vi "ReversedEngineering UpdateAttributes.vi"(1 "ClassPath/LvClassRef":variant, 2 "NewAttributes":string="Sträng:STRING\nMittCluster:CLUSTER", 3 "ClassInfo":cluster{"ClassNamn":string, "ClassPath":path}[](array[cluster]), 5 "error in (no error)":errorcluster, 6 "Don't Prompt (False)":bool, 7 "Attributes":T1[](array[typedef]), 8 "Stereotype":string) -> (18 "Cancel":bool=TRUE, 19 "error out":errorcluster)   [LabVIEW 2012] (continued)
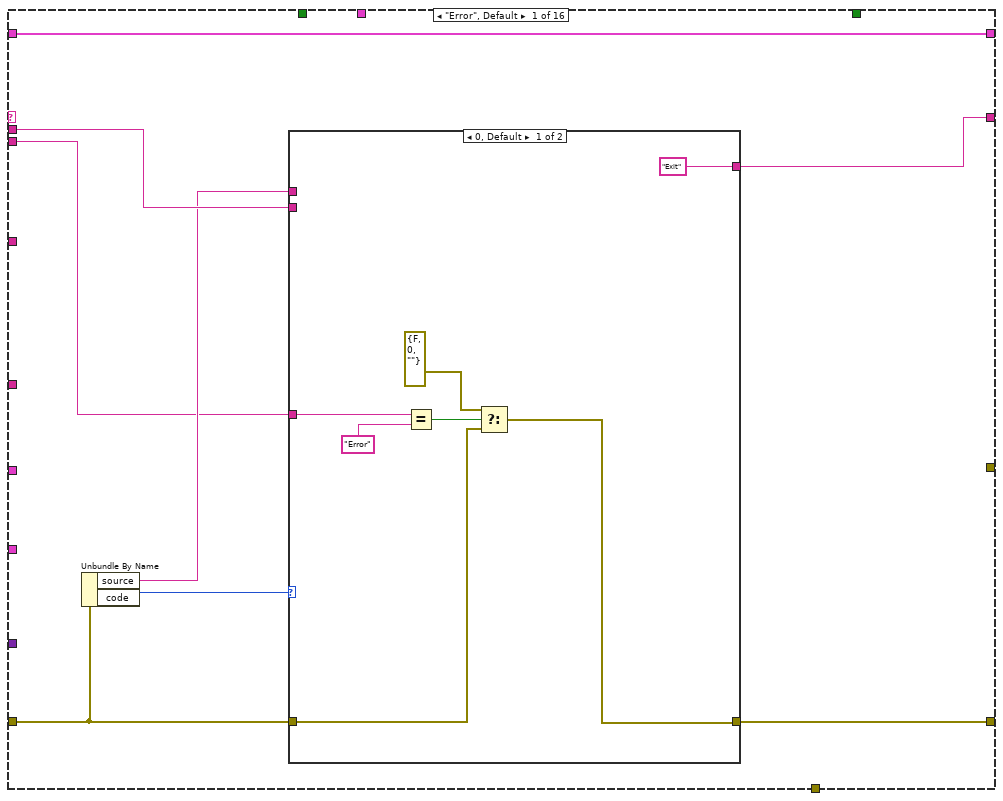
[diagram p3: hidden frame]
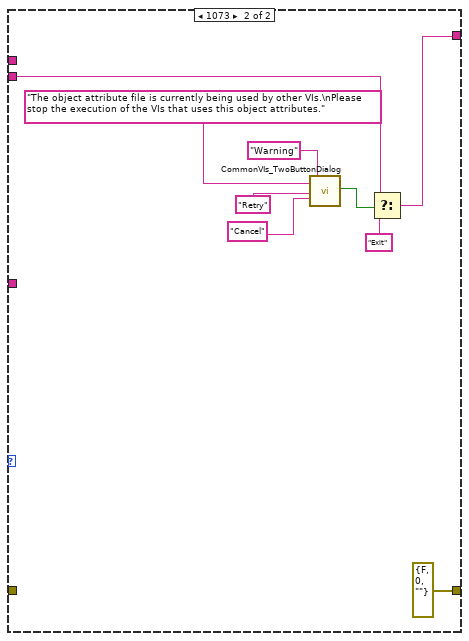
[diagram p4: hidden frame]
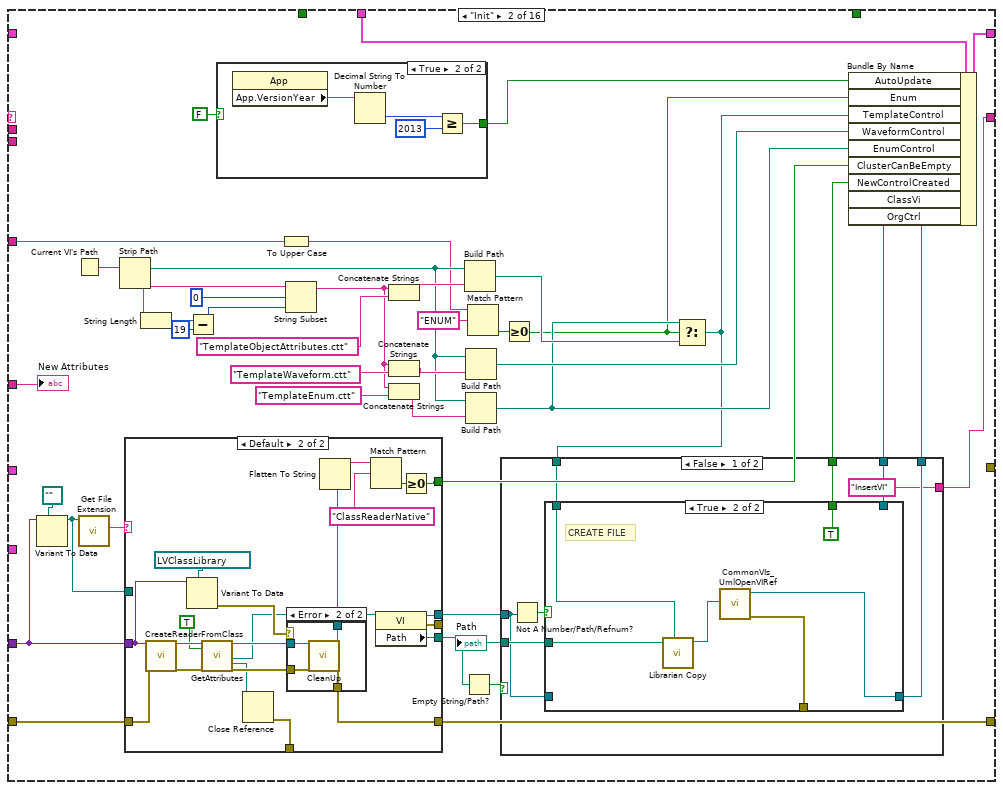
[diagram p5: hidden frame]
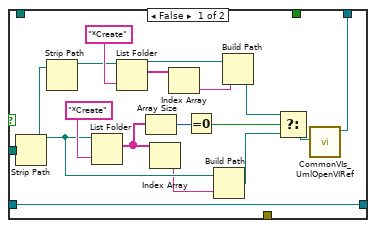
[diagram p7: hidden frame]
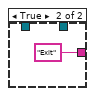
[diagram p8: hidden frame]
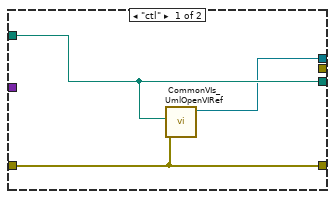
[diagram p9: hidden frame]
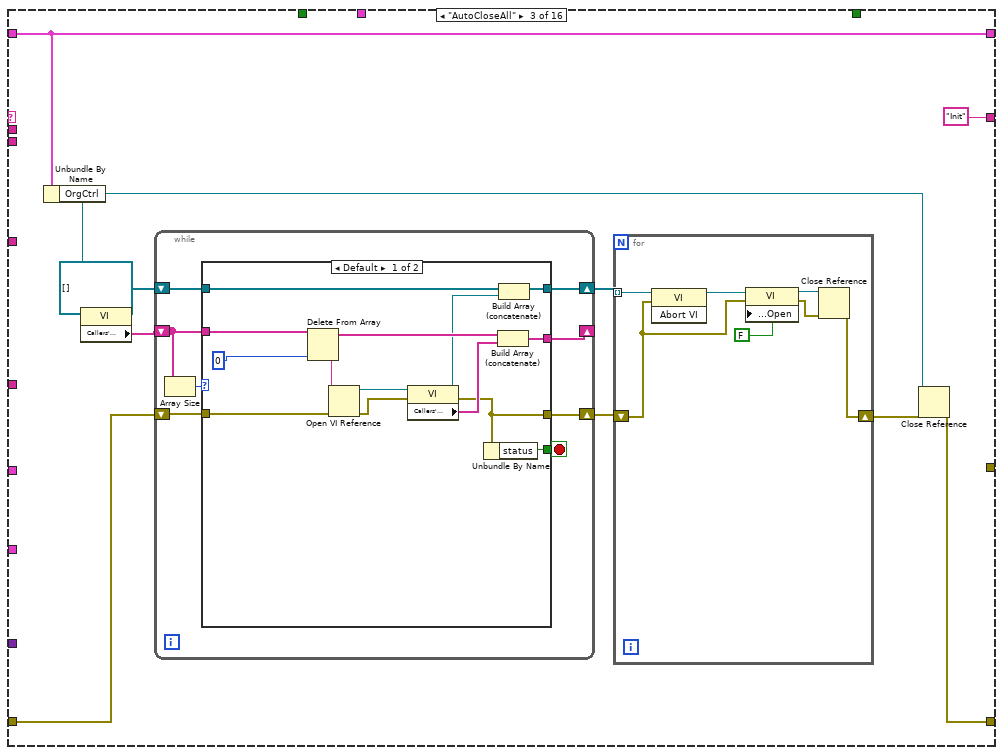
[diagram p11: hidden frame]
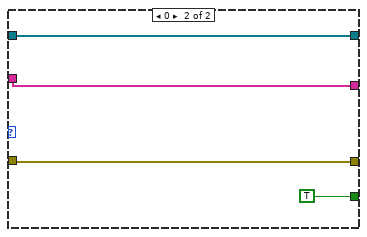
[diagram p12: hidden frame]
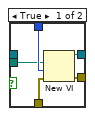
[diagram p13: hidden frame]
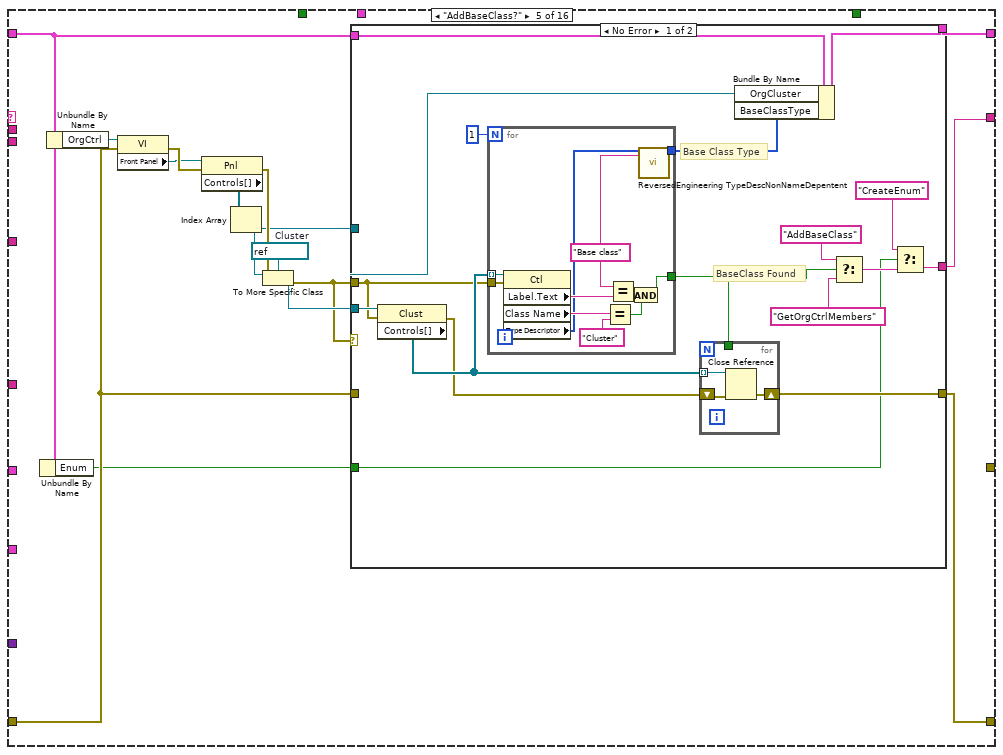
[diagram p15: hidden frame]
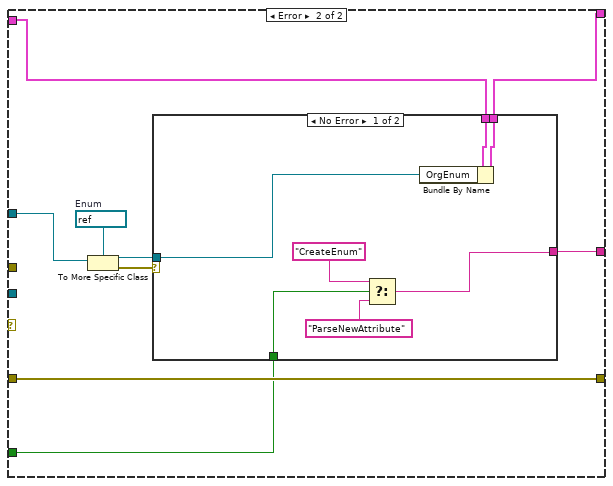
[diagram p16: hidden frame]
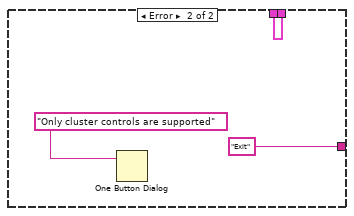
[diagram p17: hidden frame]
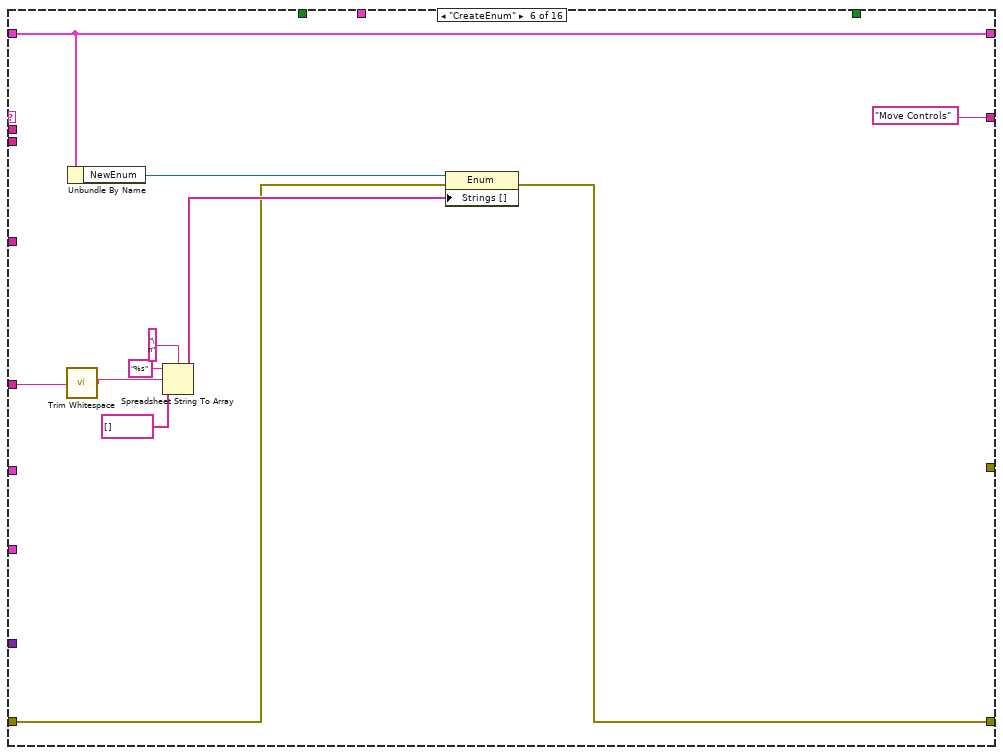
[diagram p18: hidden frame]
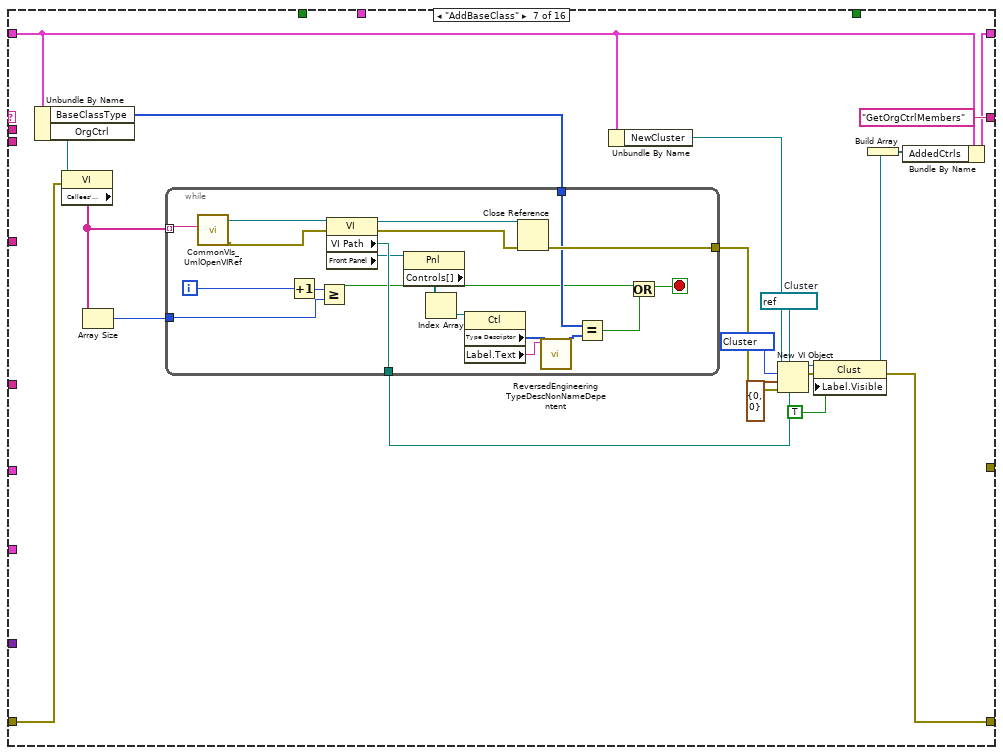
[diagram p19: hidden frame]
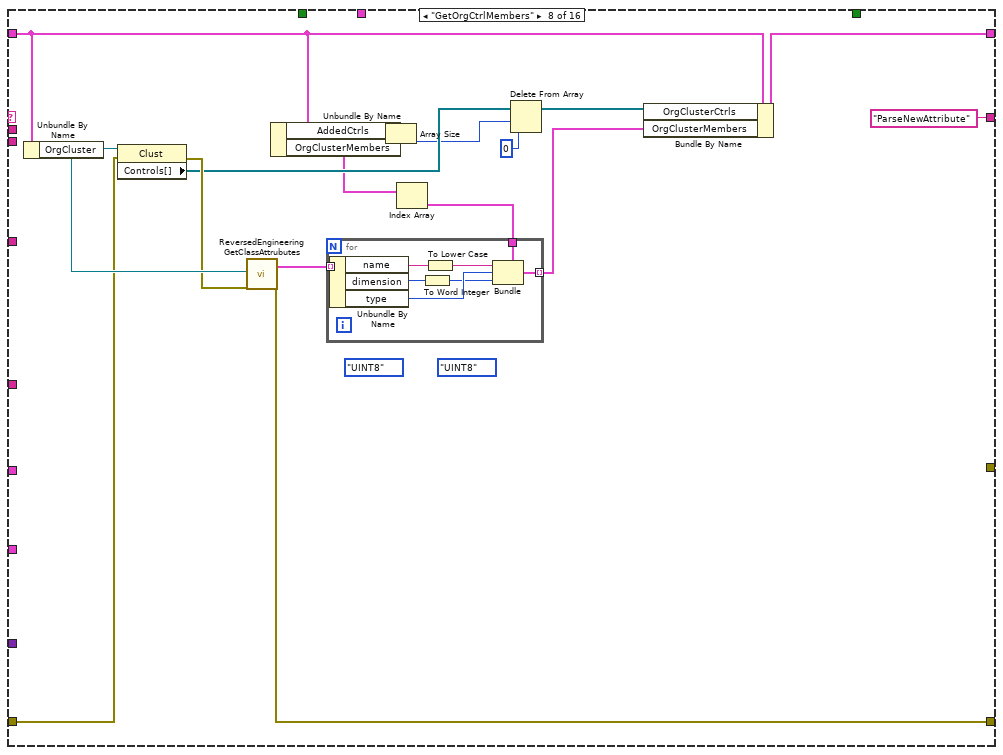
[diagram p20: hidden frame]
"Pressure Tank"=21753, "Pressure Tank 1"=3075, "Preview Queue Element"=9112, "Printable?"=1124, "Priority Queue Refnum"=3425, "Property Node"=1920, "Pulldown Menu Ring"=3061, "Push Button"=21001, "Queue Refnum"=3474, "Queue Refnum 1"=3424, "Quit LabVIEW"=1352, "Quotient & Remainder"=1056, "RT FIFO Create"=24000, "RT FIFO Delete"=24003, "RT FIFO Read"=24001, "RT FIFO Write"=24002, "Radio Buttons"=22001, "Raised Box"=3637, "Raised Box 1"=3600, "Raised Circle"=3603, "Raised Down Triangle"=3615, "Raised Frame"=3606, "Raised Left Triangle"=3612, "Raised Right Triangle"=3613, "Raised Rounded Box"=3609, "Raised Up Triangle"=3614, "Random Number (0-1)"=1070, "RcvRespMsg"=1972, "Re/Im To Complex"=1046, "Re/Im To Polar"=23060, "Read Datalog"=8069, "Read Device"=1432, "Read File"=1407, "Read from Binary File"=8051, "Read from Text File"=8070, "ReadStatus"=1973, "Receive"=1974, "ReceiveSetup"=1975, "Recessed Box"=3601, "Recessed Circle"=3604, "Recessed Down Triangle"=3619, "Recessed Frame"=3607, "Recessed Left Triangle"=3616, "Recessed Menu Ring"=3019, "Recessed Right Triangle"=3617, "Recessed Rounded Box"=3610, "Recessed Up Triangle"=3618, "Reciprocal"=1059, "Reciprocal Of Pi"=23507, "Reciprocal Of e"=23511, "Rectangular Stop Button"=3128, "Refnum to Path"=1424, "Refnum to Session"=2306, "Register Event Callback"=2078, "Register For Events"=2065, "Register Session"=2319, "Release Notifier"=9102, "Release Queue"=9109, "Replace Array Subset"=3910, "Replace Substring"=3913, "Request Deallocation"=1610, "ResetSys"=1976, "Reshape Array"=2055, "Reverse 1D Array"=1900, "Reverse String"=1537, "Right Arrow"=3825, "Right Bow Valve"=21765, "Right Bow Valve 1"=3805, "Right Bow Valve 2"=3705, "Right Down Elbow"=3717, "Right Down Elbow 1"=3817, "Right Pump"=3819, "Right Pump 1"=3719, "Right Rect Valve"=3704, "Right Rect Valve 1"=3804, "Right Rect Valve 2"=21764, "Right Tee"=3815, "Right Tee 1"=3715, "Right Up Elbow"=3714, "Right Up Elbow 1"=3814, "Ring Constant"=2008, "Rocker"=21002, "Rotary Feeder"=3830, "Rotate"=1082, "Rotate 1D Array"=1906, "Rotate Left With Carry"=1606, "Rotate Right With Carry"=1607, "Rotate String"=1536, "Round Button"=3100, "Round LED"=3120, "Round LED 1"=21012, "Round Light"=3104, "Round Push Button"=3112, "Round Push Button 2"=3118, "Round Radio Button"=3106, "Round Stop Button"=3127, "Round To +Infinity"=1076, "Round To -Infinity"=1075, "Round To Nearest"=1055, "Rydberg Constant (1/m)"=23521, "Scale By Power Of 2"=1074, "Scan From File"=2082, "Scan From String"=2080, "Scan String For Tokens"=8101, "Scan Value"=1534, "Search 1D Array"=1901, "Search and Replace String"=3914, "Search/Split String"=1538, "Secant"=1203, "Seconds To Date/Time"=1309, "Seek"=1409, "Select"=1516, "Send"=1977, "Send Notification"=9104, "SendCmds"=1978, "SendDataBytes"=1979, "SendIFC"=1980, "SendLLO"=1982, "SendList"=1981, "SendSetup"=1983, "Session to Refnum"=2307, "Set Datalog Position"=8072, "Set File Position"=8073, "Set File Size"=8074, "Set Menu Item Info"=9006, "Set Number of Records"=8075, "Set Occurrence"=1702, "Set Permissions"=8076, "Set Type and Creator"=8077, "Set Variant Attribute"=8204, "Set Waveform Attribute"=8207, "SetRWLS"=1984, "SetTimeOut"=1985, "Shared Variable Constant"=3473, "Shared Variable Control"=21814, "Shared Variable Control 1"=3472, "Shared Variable to String"=1831, "Sign"=1049, "Simple Horizontal Slide"=3003, "Simple Numeric"=3029, "Simple Numeric 1"=2900, "Simple String"=2115, "Simple Vertical Slide"=3002, "Simulation Loop"=2099, "Sinc"=1227, "Sine"=1200, "Sine & Cosine"=1220, "Size Handle"=1603, "Slide Switch"=21011, "Sort 1D Array"=1120, "Sort Array of String, Sort Array of String 1"=23065, "Speed Of Light In Vacuum (m/sec)"=23518, "Split 1D Array"=1908, "Split Button"=21020, "Split Number"=1170, "Split Signals"=2351, "Spreadsheet String To Array"=1539, "Square"=23059, "Square Button"=3101, "Square LED"=3121, "Square LED 1"=21013, "Square Light"=3105, "Square Push Button"=3113, "Square Push Button 2"=3119, "Square Radio Button"=3107, "Square Root"=1060, "Stacked Sequence Structure"=2000, "State Diagram"=2051, "Static VI Reference"=2084, "Stop"=1350, "Stop Button"=21230, "String Constant"=2007, "String Control"=21701, "String Control 1"=3200, "String Indicator"=21702, "String Indicator 1"=3201, "String Length"=1502, "String Subset"=1503, "String To Byte Array"=1608, "String To IP"=1711, "String To Path"=1078, "String to Shared Variable"=1830, "Strip Path"=1420, "SubPanel"=21810, "SubPanel (Classic)"=21811, "Subtract"=3916, "Subtract 1"=1051, "Swap Bytes"=1162, "Swap Values"=2401, "Swap Vector Element"=1912, "Swap Words"=1163, "System Button"=3130, "System Cancel Button"=3131, "System Checkbox"=3132, "System Chiseled Line"=3632, "System Colored Rectangle"=3625, "System Combo Box"=21917, "System Enum"=3062, "System Horizontal Pointer Slide"=21902, "System Horizontal Progress Bar"=21910, "System Horizontal Slide"=21904, "System Label"=21961, "System Listbox"=21805, "System Multicolumn Listbox"=21798, "System Numeric"=21919, "System Path Control"=21922, "System Pict Ring"=21925, "System Radio Button"=3133, "System Radio Buttons"=22002, "System Recessed Frame"=3624, "System Ring"=3060, "System Spin Control"=21900, "System String"=21920, "System Tab Control"=3331, "System Table"=21797, "System Time Stamp"=21967, "System Tree"=21794, "System Vertical Pointer Slide"=21901, "System Vertical Progress Bar"=21909, "System Vertical Slide"=21903, "TCP Close Connection"=1713, "TCP Create Listener"=1717, "TCP Flattened Read"=1718, "TCP Flattened Write"=1719, "TCP Flex Read"=1720, "TCP Flex Write"=1721, "TCP Network Connection Refnum"=3407, "TCP Open Connection"=1715, "TCP Read"=1716, "TCP Wait On Listener"=1712, "TCP Write"=1714, "TDMS Close"=2013, "TDMS Defragment"=2019, "TDMS File"=3477, "TDMS Flush"=2017, "TDMS Get Properties"=2015, "TDMS List Contents"=2016, "TDMS Open"=2012, "TDMS Read"=2011, "TDMS Set Properties"=2014, "TDMS Write"=2010, "TDMS Write IP"=2018, "Tab Constant"=23502, "Tab Control"=3332, "Tab Control 1"=3330, "Table"=21796, "Table 1"=21790, "Tag Attribute Ring"=2063, "Tag Constant"=2089, "Tag Control"=3302, "Tag Control 1"=21742, "Tag Indicator"=3303, "Tag Indicator 1"=21743, "Tangent"=1202, "Tank"=21006, "Tank 1"=3020, "Temporary Directory"=1435, "TestSRQ"=1986, "TestSys"=1987, "Text & Pict Ring"=21603, "Text & Pict Ring 1"=3016, "Text Button"=21015, "Text Ring"=21601, "Text Ring 1"=3014, "Text to UTF-8"=23066, "Thermometer"=21007, "Thermometer 1"=3021, "Thick Chiseled Line"=3630, "Thick Line"=3629, "Thick Line with Arrow"=3631, "Thick Lowered Box"=3635, "Thin Chiseled Line"=3627, "Thin Line"=3626, "Thin Line with Arrow"=3628, "Threshold 1D Array"=1909, "Tick Count (ms)"=1300, "Time Stamp Constant"=2068, "Time Stamp Control"=5555, "Time Stamp Control 1"=21913, "Time Stamp Indicator"=5556, "Time Stamp Indicator 1"=21914, "Timed Loop"=5570, "Timed Sequence"=5573, "To Byte Integer"=1140, "To Double Precision Complex"=1152, "To Double Precision Float"=1147, "To Extended Precision Complex"=1154, "To Extended Precision Float"=1149, "To Long Integer"=1142, "To Lower Case"=1189, "To More Generic Class"=8017, "To More Specific Class"=8016, "To OLE Variant"=8002, "To Quad Integer"=1155, "To Single Precision Complex"=1151, "To Single Precision Float"=1146, "To Time Stamp"=5560, "To Unsigned Byte Integer"=1143, "To Unsigned Long Integer"=1145, "To Unsigned Quad Integer"=1156, "To Unsigned Word Integer"=1144, "To Upper Case"=1188, "To Variant"=8201, "To Word Integer"=1141, "Traditional DAQ Channel"=21733, "Traditional DAQ Channel 1"=3320, "Traditional DAQ Channel 2"=2085, "Transpose 2D Array"=1902, "Tree"=21819, "Tree 1"=21793, "Trigger"=1988, "TriggerList"=1989, "Two Button Dialog"=1341, "Type Cast"=1166, "Type and Creator"=1434, "UDP Close"=1726, "UDP Multicast Open"=1727, "UDP Network Connection Refnum"=3418, "UDP Open"=1723, "UDP Read"=1724, "UDP Write"=1725, "UTF-8 to Text"=23067, "Unbundle"=2048, "Unbundle By Name"=2058, "Unflatten From String"=1165, "Unflatten From XML"=8401, "Unpackage Matrix"=23000, "Unregister For Events"=2076, "Unregister Session"=2320, "Up Arrow"=3823, "Up Bow Valve"=21763, "Up Bow Valve 1"=3803, "Up Bow Valve 2"=3703, "Up Rect Valve"=3702, "Up Rect Valve 1"=3802, "Up Rect Valve 2"=21762, "Up Tee"=3712, "Up Tee 1"=3812, "User Defined Refnum"=3428, "User Defined Refnum Tag"=3429, "User Defined Refnum Tag 1"=21745, "User Defined Refnum Tag Flatten"=3454, "User Defined Refnum Tag Flatten 1"=21747, "User Defined Tag"=2114, "User Defined Tag 1"=21749, "User Item"=3506, "VI Library"=1425, "VI Refnum"=3422, "VI Server Reference"=2091, "VISA Assert Interrupt Signal"=2309, "VISA Assert Trigger"=1929, "VISA Assert Utility Signal"=2310, "VISA Clear"=1927, "VISA Close"=1922, "VISA Disable Event"=1940, "VISA Discard Events"=1941, "VISA Enable Event"=1942, "VISA Find Resource"=1923, "VISA Flush I/O Buffer"=2302, "VISA GPIB Command"=2315, "VISA GPIB Control ATN"=2316, "VISA GPIB Control REN"=2304, "VISA GPIB Pass Control"=2317, "VISA GPIB Send IFC"=2318, "VISA In 16"=1930, "VISA In 32"=1944, "VISA In 8"=1936, "VISA Lock"=1993, "VISA Map Address"=1932, "VISA Map Trigger"=2311, "VISA Memory Allocation"=1997, "VISA Memory Free"=1998, "VISA Move"=2303, "VISA Move In 16"=1948, "VISA Move In 32"=1991, "VISA Move In 8"=1946, "VISA Move Out 16"=1949, "VISA Move Out 32"=1992, "VISA Move Out 8"=1947, "VISA Open"=2308, "VISA Out 16"=1931, "VISA Out 32"=1945, "VISA Out 8"=1937, "VISA Peek 16"=1934, "VISA Peek 32"=1995, "VISA Peek 8"=1938, "VISA Poke 16"=1935, "VISA Poke 32"=1996, "VISA Poke 8"=1939, "VISA Read"=1925, "VISA Read STB"=1928, "VISA Read To File"=2313, "VISA Refnum to Session"=2300, "VISA Resource Name"=21737, "VISA Resource Name 1"=3421, "VISA Set I/O Buffer Size"=2301, "VISA Status Description"=1924, "VISA USB Control In"=2086, "VISA USB Control Out"=2087, "VISA Unlock"=1994, "VISA Unmap Address"=1933, "VISA Unmap Trigger"=2312, "VISA VXI Cmd or Query"=2305, "VISA Wait on Event"=1943, "VISA Write"=1926, "VISA Write From File"=2314, "VISA resource name"=3409, "Variant"=3310, "Variant To Data"=8003, "Variant To Flattened String"=8203, "Vert Line"=3822, "Vert Pipe"=3716, "Vert Pipe 1"=3816, "Vert Rocker"=21740, "Vertical Fill Slide"=21014, "Vertical Fill Slide 1"=3009, "Vertical Graduated Bar"=21107, "Vertical Pointer Slide"=21017, "Vertical Pointer Slide 1"=3007, "Vertical Progress Bar"=21104, "Vertical Scrollbar"=21111, "Vertical Slide"=3004, "Vertical Slide Switch"=21741, "Vertical Slide Switch 1"=3115, "Vertical Smooth Box"=3634, "Vertical Splitter Bar"=21860, "Vertical Splitter Bar (Classic)"=21862, "Vertical Splitter Bar (System)"=21864, "Vertical Switch"=3109, "Vertical Toggle Switch"=21005, "Vertical Toggle Switch 1"=3111, "Volume Info"=1414, "Wait (ms)"=1302, "Wait For Activity"=1722, "Wait For Front Panel Activity"=1328, "Wait Until Next ms Multiple"=1327, "Wait for GPIB RQS"=1952, "Wait on Notification"=9105, "Wait on Notification from Multiple"=9106, "Wait on Occurrence"=1701, "WaitSRQ"=1990, "Waveform Chart"=3501, "Waveform Chart 1"=21717, "Waveform Chart 2"=21010, "Waveform Graph"=21703, "Waveform Graph 1"=3504, "While Loop"=2003, "While Loop 1"=2352, "White Space?"=1125, "Write Datalog"=8079, "Write Device"=1431, "Write File"=1408, "Write to Binary File"=8078, "Write to Text File"=8080, "XY Graph"=3500, "XY Graph 1"=21716, "Xmath Script Node"=9022, "Y-th root of X"=23062]
                      (unwired) refnum<vi> refnum  # LVObjectRefNum
                      n229 = New VI Object(vi object class=w701, owner refnum=w707, style=w702, position/next to=w706, 8:w704) -> (object refnum=w703:refnum<vi>, 0:w705:errorcluster)  [unwired: 3 out]
                    }
                  }
                  n230 = case shown="0, Default" w527 {
                    tunnel: w530 -> [w540 w543]
                    tunnel: [w540 w542] -> w528
                    tunnel: w526 -> [_ w542]
                    tunnel: [_ w541] -> _
                    frame 0, Default {
                    }
                    frame 1.. {
                      n231 = Close Reference(reference=w543) -> (error out=w541:errorcluster)  [unwired: 1 in]
                    }
                  }
                }
                frame True {
                  # "Control exists, no change, just copy"
                  n232 = Index Array(array=w746, index=w711) -> (element=w724:refnum<vi>)
                  n233 = property class="Ctl"(reference=w744, error in=w727) -> ("Position:Top"=w743:i32, "Bounds:Height"=w742:u32)  [unwired: 2 out]
                  n234 = property on="Panel" class="VI"(reference=w733, error in=w727) -> (error out=w734:errorcluster, "Front Panel"=w728:refnum<vi>)  [unwired: 1 out]
                  n235 = Build Array (concatenate)(w712, w711) -> (w710:i32[])
                  n236 = Add(x=w743, y=w742) -> (x+y=w741:u32)
                  n237 = property on="Select" class="Ctl"(reference=w724, error in=w734, "Selected"=TRUE) -> (error out=w735:errorcluster)  [unwired: 1 out]
                  n238 = Increment(x=w741) -> (x+1=w740:u32)
                  n239 = Bundle("element"=u32 0, w740) -> (w720:cluster{"element":u32, u32})  [unwired: 1 out]
                  n240 = invoke on="Copy" class="Pnl" method="Copy Selection"(reference=w728, error in=w735) -> (reference out=w737:refnum<vi>, error out=w736:errorcluster)  [unwired: 1 in, 1 out]
                  n241 = Close Reference(reference=w737, error in (no error)=w736) -> (error out=w726:errorcluster)
                  n242 = property on="Select" class="Ctl"(reference=w724, error in=w726, "Selected"=FALSE) -> (error out=w725:errorcluster)  [unwired: 1 out]
                  n243 = property on="Panel" class="VI"(reference=w723, error in=w725) -> (error out=w745:errorcluster, "Front Panel"=w719:refnum<vi>)  [unwired: 1 out]
                  n244 = invoke class="Pnl" method="Paste Selection"(reference=w719, error in=w745, "Pos"=cluster{"Left":i32, "Top":i32} {"Left"=50, "Top"=50}) -> (reference out=w716:refnum<vi>, error out=w715:errorcluster)  [unwired: 2 in, 3 out]
                  n245 = property on="Panel" class="Pnl"(reference=w716, error in=w715) -> (reference out=w730:refnum<vi>, error out=w714:errorcluster, "Controls[]"=w731:refnum<vi>[])
                  n246 = Delete From Array(array=w731) -> (deleted portion=w709:refnum<vi>, array with subset deleted=w718:refnum<vi>[])  [unwired: 2 in]
                  n247 = invoke class="Ctl" method="Move"(reference=w709, error in=w714, "position"=w720, "owner"=w721) -> (reference out=w708:refnum<vi>, error out=w713:errorcluster)  [unwired: 2 in, 4 out]
                  n248 = invoke on="Paste" class="Ctl" method="Update Typedef"(reference=w709) -> ()  [unwired: 2 in, 3 out]
                  n249 = Close Reference(reference=w730, error in (no error)=w713) -> (error out=w729:errorcluster)
                  n250 = for {
                    tunnel: w718 -> [w747] mode=indexing
                    tunnel: w708 -> [_]
                    n251 = Close Reference(reference=w747) -> ()  [unwired: 1 in, 1 out]
                  }
                  n252 = invoke on="EmptyClip" class="App" method="Clipboard.Empty"(error in=w729) -> (error out=w732:errorcluster)  [unwired: 2 in, 2 out]
                }
              }
              n253 = property class="Ctl"(reference=w512, error in=w520, "Label.Text"=w492, "Auto-Update From Typedef"=TRUE ("Label.Visible")) -> (reference out=w522:refnum<vi>, error out=w521:errorcluster)
              n254 = property class="Ctl"(reference=w522, error in=w521, "Label.Text"=w492, "Label.Visible"=TRUE) -> (reference out=w523:refnum<vi>, error out=w519:errorcluster)
            }
            n255 = Array Size(array=w466) -> (size(s)=w465:i32)
            n256 = Array Size(array=w467) -> (size(s)=w464:i32)
            n257 = Equal?(x=w465, y=w464) -> (x = y?=w463:bool)
            n258 = And Array Elements(Boolean array=w467) -> (logical AND=w468:bool)
            n259 = And(x=w463, y=w468) -> (x .and. y?=w462:bool)
            n260 = Build Array (concatenate)(w482, w480) -> (w481:refnum<vi>[])
            n261 = Bundle By Name(cluster=w471, "NoUpdate"=w462, "AddedCtrls"=w481) -> (w483:T4)
          }
          frame "Move Controls" {
            n262 = Unbundle By Name(w753) -> ("NewCtrl"=w764:refnum<vi>, "NewCluster"=w763:refnum<vi>, "OrgCtrl"=w760:refnum<vi>, "OrgCluster"=w761:refnum<vi>, "NewEnum"=w754:refnum<vi>)
            n263 = property class="VI"(reference=w760) -> ("Front Panel Window:Origin"=w762:T12)  [unwired: 1 in, 2 out]
            n264 = property class="VI"(reference=w764) -> ("Front Panel Window:Origin"=w755:T12)  [unwired: 1 in, 2 out]
            n265 = property class="Clust"(reference=w761, "Position"=w762) -> ()  [unwired: 1 in, 2 out]
            n266 = property class="Clust"(reference=w763, "Position"=w755) -> ()  [unwired: 1 in, 2 out]
            n267 = property class="Enum"(reference=w754, "Position"=w755) -> ()  [unwired: 1 in, 2 out]
            n268 = case shown="True" FALSE {
              tunnel: [_ w766] -> w749
              frame False {
              }
              frame True {
                n269 = property class="App"() -> ("App.VersionYear"=w769:string)  [unwired: 2 in, 2 out]
                n270 = Decimal String To Number(string=w769) -> (number=w768:i32)  [unwired: 2 in, 1 out]
                n271 = Greater Or Equal?(x=w768, y=2013) -> (x >= y?=w766:bool)
              }
            }
            n272 = Unbundle By Name(w753) -> ("NoUpdate"=w751:bool, "AutoUpdate"=w750:bool)
            n273 = Compound Arithmetic op=OR(w756, w751, w750, w749) -> (w752:bool)
            n274 = Select(t="SaveCtrl" ("y"), s=w752, f="Idle" ("y")) -> (s? t:f=w757:string)
          }
          frame "Idle" {
            n275 = call <resource>:"ContextHelp_EnteringDialog.vi"() -> ("HelpStatus"=w770:bool, "error out"=w773:errorcluster)  [unwired: 3 in, 15 out]
            n276 = Unbundle By Name(w785) -> ("NewCluster"=w784:refnum<vi>, "OrgCtrl"=w776:refnum<vi>)  [unwired: 1 out]
            n277 = call <resource>:"CommonVIs_GetFrontPanelControls.vi"("error in (no error)"=w773) -> ("Event Registration Refnum"=w772:refnum<event-registration>, "ControlRefs"=w775:refnum<vi>[])  [unwired: 1 in, 16 out]
            n278 = while {
              tunnel: [w797] -> w787
              tunnel: w776 -> [w796]
              tunnel: w772 -> [w794]
              tunnel: [w793] -> w771
              stop <- w795 stop-if-true
              n279 = event shown="[1] \"Backup\": Value Change" {
                selector: w794 -> [_ _ _ _ _ _]
                dyn-events: [_ _ _ _ _ _] -> w793
                timeout: 500 -> [_ _ _ _ _ _]
                tunnel: ["Cancel" _ _ _ _ TRUE ("Cancel")] -> w797
                tunnel: w796 -> [_ w811 _ _ _ _]
                tunnel: [TRUE _ _ _ _ TRUE] -> w795
                event "OK", "Cancel": Value Change {
                  n280 = event-data() -> ()  [unwired: 2 out]
                  n281 = case shown="True" "OK" {
                    frame False {
                    }
                    frame True {
                      n282 = call <vilib>:"Set Busy.vi"() -> ()  [unwired: 4 in, 8 out]
                    }
                  }
                }
                event "Backup": Value Change {
                  n283 = event-data() -> ()  [unwired: 2 out]
                  n284 = call <vilib>:"Dflt Data Dir.vi"() -> ("App:Default Data Directory"=w822:path)
                  n285 = Format Date/Time String(time format string (%c)="%y%m%d_%H%M%S_") -> (date/time string=w817:string)  [unwired: 2 out]
                  n286 = property class="VI"(reference=w811) -> (reference out=w813:refnum<vi>, error out=w812:errorcluster, "VI Name"=w803:string)  [unwired: 1 in]
                  n287 = Build Path(base path=w822, name or relative path="Backup") -> (appended path=w818:path)
                  n288 = Match Pattern(string=w803, regular expression=":") -> (after substring=w802:string)  [unwired: 4 out]
                  n289 = Create Folder(path (use dialog)=w818) -> (created path=w806:path)  [unwired: 1 in, 3 out]
                  n290 = Concatenate Strings(w817, w802) -> (w807:string)
                  n291 = Build Path(base path=w806, name or relative path=w807) -> (appended path=w809:path)
                  n292 = Format Into String(format string="Do you want to save a backup file\nof the original control here.\n\n%s", w809) -> (resulting string=w819:string)  [unwired: 2 in, 1 out]
                  n293 = Two Button Dialog(message=w819, 1:"No" ("F button name (\"Cancel\")"), 2:"Yes" ("T button name (\"OK\")")) -> (T button?=w810:bool)
                  n294 = case shown="False" w810 {
                    tunnel: w809 -> [_ w830]
                    tunnel: [w826 w830] -> w808
                    tunnel: w807 -> [w828 _]
                    tunnel: w806 -> [w827 _]
                    tunnel: [w825 _] -> w805
                    tunnel: "Select backup file path" ("prompt") -> [w824 _]
                    frame False {
                      (unwired) T13."new or existing file" ("select mode (2)")
                      n295 = File Dialog(5:"Save" ("button label"), 6:"*.ctl" ("default name"), 7:w824, 9:w828, 11:w827) -> (1:w825:bool, 3:w826:path)  [unwired: 1 in, 3 out]
                    }
                    frame True {
                    }
                  }
                  n296 = case shown="False" w805 {
                    tunnel: w812 -> [w836 w837]
                    tunnel: w813 -> [w832 w838]
                    tunnel: w808 -> [w835 _]
                    tunnel: [w834 w838] -> _
                    tunnel: [w833 w837] -> _
                    frame False {
                      n297 = invoke class="VI" method="Save.Instrument"(reference=w832, error in=w836, "Path to saved file"=w835, "Save a Copy"=TRUE) -> (reference out=w834:refnum<vi>, error out=w833:errorcluster)  [unwired: 2 in, 4 out]
                    }
                    frame True {
                    }
                  }
                }
                event Timeout {
                  n298 = event-data() -> ()  [unwired: 2 out]
                  n299 = property class="VI"("Front Panel Window:Is Frontmost"=TRUE) -> ()  [unwired: 2 in, 2 out]
                }
                event "Help": Value Change {
                  n300 = event-data() -> ()  [unwired: 2 out]
                  n301 = case shown="False" "Help" {
                    tunnel: [ContextHelp_HelpTexts."None(Hide)" ("HelpText") ContextHelp_HelpTexts."ReversedEngineering UpdateAttributes_AllButtons" ("HelpText")] -> w841
                    frame False {
                    }
                    frame True {
                    }
                  }
                  n302 = call <resource>:"ContextHelp_HelpTexts.vi"("HelpText (enum or string)"=w841) -> ("HelpOut"=w842:T14)  [unwired: 18 out]
                  n303 = call <resource>:"ContextHelp_SendMessageToPopUp.vi"("PopUpMessage"=w842) -> ()  [unwired: 2 in, 17 out]
                }
                event Mouse Enter {
                  n304 = event-data() -> ("CtlRef"=w846:refnum<vi>)  [unwired: 1 out]
                  n305 = local read "Help"() -> (w845:bool)
                  n306 = call <resource>:"ContextHelp_CheckHelpForControl.vi"("Ctl Refnum"=w846, "Help"=w845) -> ()  [unwired: 1 in, 17 out]
                }
                event Panel Close? {
                  n307 = event-data() -> ()  [unwired: 2 out]
                  n308 = event-data("Discard?"=TRUE) -> ()  [unwired: 1 in, 1 out]
                }
              }
            }
            n309 = property on="Help" class="Bool (strict)"("Value (Signaling)"=w770) -> ()  [unwired: 2 in, 2 out]
            n310 = property class="Clust"(reference=w784, "Auto Sizing"=u32 3) -> ("Controls[]"=w778:refnum<vi>[])  [unwired: 1 in, 2 out]
            n311 = Index Array(array=w778) -> (element=w782:refnum<vi>)  [unwired: 1 in]
            n312 = property class="Ctl"(reference=w782) -> (reference out=w781:refnum<vi>, "Position:Left"=w780:i32)  [unwired: 1 in, 1 out]
            n313 = Increment(x=w780) -> (x+1=w779:i32)
            n314 = property class="Ctl"(reference=w781, "Position:Left"=w779) -> (error out=w777:errorcluster)  [unwired: 1 in, 1 out]
            n315 = for {
              tunnel: w778 -> [w850] mode=indexing
              tunnel: w777 -> [_]
              n316 = Close Reference(reference=w850) -> ()  [unwired: 1 in, 1 out]
            }
            n317 = invoke class="VI" method="FP.Open"() -> ()  [unwired: 5 in, 5 out]
            n318 = call <resource>:"CommonVIs_CloseControlRefs.vi"("Event Registration Refnum"=w771, "ControlRefs"=w775) -> ("error out"=w774:errorcluster)  [unwired: 1 in, 16 out]
            n319 = Bundle By Name(cluster=w785, "Cancel"=w787) -> (w788:T4)
            n320 = call <resource>:"ContextHelp_LeavingDialog.vi"("error in (no error)"=w774) -> ()  [unwired: 2 in, 17 out]
            n321 = Select(t="Exit" ("y"), s=w787, f="SaveCtrl" ("y")) -> (s? t:f=w789:string)
          }
          frame "SaveCtrl" {
            n322 = Unbundle By Name(w865) -> ("NewEnum"=w859:refnum<vi>, "OrgCluster"=w863:refnum<vi>, "OrgCtrl"=w855:refnum<vi>)  [unwired: 1 out]
            n323 = stacked-sequence {
              tunnel: w858 -> [w872]
              tunnel: [w872] -> w851
              tunnel: [w871] -> _
              tunnel: [w870] -> _
              frame #0 {
                n324 = invoke on="Attribute Before" class="SubPanel" method="Remove VI"() -> (error out=w871:errorcluster)  [unwired: 3 in, 2 out]
                n325 = invoke on="Attribute After" class="SubPnl" method="Remove VI"() -> (error out=w870:errorcluster)  [unwired: 3 in, 2 out]
              }
            }
            n326 = invoke class="VI" method="FP.Open"(reference=w855, error in=w851) -> (reference out=w854:refnum<vi>)  [unwired: 3 in, 4 out]
            n327 = property class="VI"(reference=w855, error in=w851, "Front Panel Window:Origin"=cluster{"Horizontal":i16, "Vertical":i16} {"Horizontal"=0, "Vertical"=0}) -> (error out=w853:errorcluster)  [unwired: 1 out]
            n328 = property class="Clust"(reference=w863, error in=w853, "Position"=cluster{"Left":i32, "Top":i32} {"Left"=5, "Top"=5}) -> (error out=w856:errorcluster)  [unwired: 1 out]
            n329 = property class="Enum"(reference=w859, error in=w853, "Position"=cluster{"Left":i32, "Top":i32} {"Left"=5, "Top"=5}) -> (error out=w857:errorcluster)  [unwired: 1 out]
            n330 = invoke class="VI" method="CtlVIApplyChanges"(reference=w854) -> (reference out=w852:refnum<vi>)  [unwired: 2 in, 2 out]
            n331 = stacked-sequence {
              tunnel: w852 -> [w869]
              tunnel: w853 -> [w868]
              tunnel: w857 -> [_]
              tunnel: w856 -> [_]
              frame #0 {
                n332 = invoke class="VI" method="Save.Instrument"(reference=w869, error in=w868) -> (reference out=w867:refnum<vi>, error out=w866:errorcluster)  [unwired: 4 in, 4 out]
                n333 = invoke class="VI" method="FP.Close"(reference=w867, error in=w866) -> ()  [unwired: 1 in, 3 out]
              }
            }
          }
          frame "ReplaceCtrl" {
            n334 = Unbundle By Name(w925) -> ("Enum"=w897:bool, "OrgEnum"=w894:refnum<vi>, "OrgCtrl"=w909:refnum<vi>, "OrgCluster"=w889:refnum<vi>, "NewCtrl"=w932:refnum<vi>, "NewCluster"=w901:refnum<vi>, "NewEnum"=w898:refnum<vi>, "ClassVi"=w915:refnum<vi>)
            n335 = property class="Clust"(reference=w889) -> (reference out=w888:refnum<vi>, "Label.Text"=w887:string)  [unwired: 1 in, 1 out]
            n336 = property class="VI"(reference=w932, error in=w923) -> (reference out=w919:refnum<vi>, error out=w890:errorcluster, "Front Panel"=w900:refnum<vi>)
            n337 = invoke class="Enum" method="Delete"(reference=w894, error in=w890) -> (reference out=w896:refnum<vi>, error out=w891:errorcluster)  [unwired: 1 in, 1 out]
            n338 = invoke class="Clust" method="Delete"(reference=w888, error in=w890) -> (reference out=w895:refnum<vi>, error out=w892:errorcluster)  [unwired: 1 in, 1 out]
            n339 = Close Reference(reference=w895, error in (no error)=w892) -> (error out=w875:errorcluster)
            n340 = Close Reference(reference=w896, error in (no error)=w891) -> (error out=w874:errorcluster)
            n341 = case shown="No Error" w891 {
              selector: w891 -> [w937 _]
              tunnel: w892 -> [_ w938]
              tunnel: [w937 w938] -> w893
              tunnel: w875 -> [_ _]
              tunnel: w874 -> [_ _]
              frame No Error {
              }
              frame Error {
              }
            }
            n342 = case shown="False" w897 {
              tunnel: w901 -> [_ w957]
              tunnel: [w954 w958] -> w899
              tunnel: w898 -> [w953 _]
              tunnel: w893 -> [w952 w956]
              frame True {
                n343 = property class="Enum"(reference=w953, error in=w952, "Selected"=TRUE) -> (error out=w954:errorcluster)  [unwired: 1 out]
              }
              frame False {
                n344 = property class="Clust"(reference=w957, error in=w956, "Selected"=TRUE) -> (error out=w958:errorcluster)  [unwired: 1 out]
              }
            }
            n345 = invoke class="Pnl" method="Copy Selection"(reference=w900, error in=w899) -> (reference out=w926:refnum<vi>, error out=w922:errorcluster)  [unwired: 1 in, 1 out]
            n346 = Close Reference(reference=w926, error in (no error)=w922) -> (error out=w921:errorcluster)
            n347 = property class="VI"(reference=w909, error in=w921) -> (error out=w930:errorcluster, "Front Panel"=w931:refnum<vi>)  [unwired: 1 out]
            n348 = invoke class="Pnl" method="Paste Selection"(reference=w931, error in=w930, "Pos"=cluster{"Left":i32, "Top":i32} {"Left"=20, "Top"=40}) -> (reference out=w927:refnum<vi>, error out=w928:errorcluster)  [unwired: 2 in, 3 out]
            n349 = Close Reference(reference=w927, error in (no error)=w928) -> (error out=w918:errorcluster)
            n350 = invoke class="App" method="Clipboard.Empty"(error in=w918) -> (error out=w904:errorcluster)  [unwired: 2 in, 2 out]
            n351 = property class="VI"(reference=w909, error in=w904) -> (reference out=w908:refnum<vi>, error out=w913:errorcluster, "Front Panel"=w910:refnum<vi>)
            n352 = property class="Pnl"(reference=w910, error in=w913) -> (reference out=w905:refnum<vi>, error out=w912:errorcluster, "Controls[]"=w907:refnum<vi>[])
            n353 = Index Array(array=w907) -> (element=w911:refnum<vi>)  [unwired: 1 in]
            n354 = case shown="False" w897 {
              tunnel: w912 -> [w942 w951]
              tunnel: w911 -> [w949 _]
              tunnel: [w942 w951] -> w902
              tunnel: w887 -> [w939 _]
              frame False {
                w950 = refnum<vi> refnum  # Cluster
                n355 = To More Specific Class(target class=w950, reference=w949, error in=w942) -> (specific class reference=w948:refnum<vi>, error out=w943:errorcluster)
                n356 = property class="Clust"(reference=w948, error in=w943, "Auto Sizing"=u32 0) -> (reference out=w946:refnum<vi>, error out=w945:errorcluster)
                n357 = property class="Clust"(reference=w946, error in=w945, "Auto Sizing"=u32 3) -> (reference out=w941:refnum<vi>, error out=w940:errorcluster)
                n358 = property class="Clust"(reference=w941, error in=w940, "Label.Text"=w939) -> ()  [unwired: 2 out]
              }
              frame True {
              }
            }
            n359 = Select(t=w904, s=w902, f=w902) -> (s? t:f=w903:errorcluster)
            n360 = invoke class="VI" method="Save.Instrument"(reference=w908, error in=w903) -> (reference out=w880:refnum<vi>, error out=w879:errorcluster)  [unwired: 4 in, 4 out]
            n361 = property class="VI"(reference=w880, error in=w879) -> (reference out=w877:refnum<vi>, error out=w882:errorcluster, "Library"=w886:refnum<vi>)
            n362 = To More Specific Class(target class=refnum<vi> refnum ("ClassRefIn"), reference=w886, error in=w882) -> (specific class reference=w884:refnum<vi>, error out=w883:errorcluster)
            n363 = for {
              tunnel: w907 -> [w962] mode=indexing
              shift-right: [w960] -> w906
              shift-left: w879 -> [w961]
              n364 = Close Reference(reference=w962, error in (no error)=w961) -> (error out=w960:errorcluster)
            }
            n365 = case shown="Error" w883 {
              selector: w883 -> [w934 _]
              tunnel: w884 -> [w935 w936]
              tunnel: [w933 w936] -> w881
              frame No Error {
                n366 = call <resource>:"GDSLvClass_SaveEverythingInClass.vi"("ClassRefIn"=w935, "error in"=w934) -> ("ClassRefOut"=w933:refnum<vi>)  [unwired: 1 in, 16 out]
              }
              frame Error {
              }
            }
            n367 = Close Reference(reference=w905, error in (no error)=w906) -> (error out=w878:errorcluster)
            n368 = Close Reference(reference=w881, error in (no error)=w878) -> (error out=w876:errorcluster)
            n369 = Close Reference(reference=w877, error in (no error)=w878) -> (error out=w920:errorcluster)
            n370 = Close Reference(reference=w919, error in (no error)=w920) -> (error out=w914:errorcluster)
            n371 = invoke class="VI" method="Save.Instrument"(reference=w915, error in=w914) -> (reference out=w916:refnum<vi>, error out=w917:errorcluster)  [unwired: 4 in, 4 out]
            n372 = Close Reference(reference=w916, error in (no error)=w917) -> (error out=w873:errorcluster)
          }
          frame "AddToProject?" {
            n373 = Unbundle By Name(w966) -> ("NewControlCreated"=w965:bool)
            n374 = case shown="True" w965 {
              tunnel: w964 -> [w968 w973]
              tunnel: [w968 w969] -> w963
              frame False {
              }
              frame True {
                n375 = call <resource>:"CommonVIs_UmlOpenVIRef.vi"("error in"=w973) -> ("error out"=w975:errorcluster, "ProjectNameOut"=w974:string)  [unwired: 3 in, 6 out]
                n376 = call <resource>:"GDSProject_GetProjects.vi"("GetProjectRefByName"=w974, "error in (no error)"=w975) -> ("Project Refnum"=w972:refnum<vi>, "error out"=w970:errorcluster)  [unwired: 1 in, 15 out]
                n377 = Not A Number/Path/Refnum?(number/path/refnum=w972) -> (NaN/Path/Refnum?=w971:bool)
                n378 = case shown="True" w971 {
                  tunnel: w972 -> [w1005 _]
                  tunnel: w970 -> [w1001 w1024]
                  tunnel: [w979 w1024] -> w969
                  tunnel: [w980 _] -> _
                  frame False {
                    w991 = refnum<vi> refnum  # LVClassLibrary
                    n379 = property class="Project"(reference=w1005, error in=w1001) -> (reference out=w988:refnum<vi>, error out=w1000:errorcluster, "My Computer"=w1003:refnum<vi>)
                    n380 = local read "Path"() -> (w994:path)
                    n381 = invoke class="TargetItem" method="Get All Descendents"(reference=w1003, error in=w1000, "Type"="lvclass") -> (reference out=w993:refnum<vi>, error out=w976:errorcluster, "All Descendents"=w1002:refnum<vi>[])  [unwired: 4 in, 4 out]
                    n382 = Strip Path(path=w994) -> (stripped path=w999:path)  [unwired: 1 out]
                    n383 = for {
                      tunnel: w1002 -> [w1023] mode=indexing
                      tunnel: w999 -> [w1020]
                      tunnel: [w1019] -> w998 mode=indexing
                      tunnel: [w1018] -> w978 mode=indexing
                      n384 = property class="ProjectItem"(reference=w1023) -> (reference out=w1018:refnum<vi>, "Path"=w1022:path)  [unwired: 1 in, 1 out]
                      n385 = Strip Path(path=w1022) -> (stripped path=w1021:path)  [unwired: 1 out]
                      n386 = call <vilib>:"Compare Two Paths.vi"("Path 2"=w1020, "Path 1"=w1021) -> ("Path 2 Relative to Path 1?"=w1019:bool)  [unwired: 1 in, 8 out]
                    }
                    n387 = Search 1D Array(1D array=w998, element=TRUE) -> (index of element=w996:i32)  [unwired: 1 out]
                    n388 = case shown="0, Default" w996 {
                      selector: w996 -> [w1015 _]
                      tunnel: w978 -> [w1016 _]
                      tunnel: [w1014 w1017] -> w995
                      tunnel: w993 -> [_ w1017]
                      frame 0, Default {
                        n389 = Index Array(array=w1016, index=w1015) -> (element=w1014:refnum<vi>)
                      }
                      frame -1 {
                      }
                    }
                    n390 = invoke class="ProjectItem" method="AddFile"(reference=w995, error in=w976, "Path"=w994) -> (reference out=w992:refnum<vi>, error out=w977:errorcluster, "AddFile"=w986:refnum<vi>)  [unwired: 1 in, 1 out]
                    n391 = property class="ProjectItem"(reference=w986) -> (reference out=w981:refnum<vi>, "Reference"=w985:refnum<vi>)  [unwired: 1 in, 1 out]
                    n392 = To More Specific Class(target class=w991, reference=w992, error in=w977) -> (specific class reference=w989:refnum<vi>, error out=w990:errorcluster)
                    n393 = invoke class="VI" method="Save.Instrument"(reference=w985) -> (reference out=w984:refnum<vi>, error out=w983:errorcluster)  [unwired: 5 in, 4 out]
                    n394 = case shown="Error" w990 {
                      tunnel: w989 -> [w1012 _]
                      tunnel: [w1011 w1013] -> w987
                      tunnel: w976 -> [_ w1013]
                      frame No Error {
                        n395 = invoke class="LVClassLibrary" method="Save"(reference=w1012) -> (error out=w1011:errorcluster)  [unwired: 3 in, 3 out]
                      }
                      frame Error {
                      }
                    }
                    n396 = Close Reference(reference=w984, error in (no error)=w983) -> (error out=w982:errorcluster)
                    n397 = stacked-sequence {
                      tunnel: w993 -> [w1010]
                      tunnel: [w1006] -> w979
                      tunnel: w988 -> [w1007]
                      tunnel: w987 -> [w1006]
                      frame #0 {
                        n398 = invoke class="Project" method="Save"(reference=w1007) -> (reference out=w1008:refnum<vi>, error out=w1009:errorcluster)  [unwired: 3 in, 2 out]
                        n399 = Close Reference(reference=w1010) -> ()  [unwired: 1 in, 1 out]
                        n400 = Close Reference(reference=w1008, error in (no error)=w1009) -> ()  [unwired: 1 out]
                      }
                    }
                    n401 = Close Reference(reference=w978, error in (no error)=w979) -> ()  [unwired: 1 out]
                    n402 = Close Reference(reference=w981, error in (no error)=w982) -> (error out=w980:errorcluster)
                  }
                  frame True {
                  }
                }
              }
            }
          }
        }
        n403 = Select(t="Error", s=w52, f=w51) -> (s? t:f=w53:string)
        n404 = Equal?(x=w51, y="Exit") -> (x = y?=w49:bool)
      }
    }
    frame Error {
    }
  }
  "error out" <- w22
  n405 = Unbundle By Name(w27) -> ("ClassVi"=w11:refnum<vi>, "NewCtrl"=w12:refnum<vi>, "NewCluster"=w13:refnum<vi>, "NewEnum"=w14:refnum<vi>, "OrgEnum"=w15:refnum<vi>, "AddedCtrls"=w4:refnum<vi>[], "OrgCtrl"=w26:refnum<vi>, "OrgCluster"=w23:refnum<vi>, "Cancel"=w19:bool, "NewControlCreated"=w18:bool)
  n406 = And(x=w19, y=w18) -> (x .and. y?=w17:bool)
  n407 = case shown="True" w17 {
    tunnel: [_ w1026] -> _
    frame False {
    }
    frame True {
      n408 = local read "Path"() -> (w1027:path)
      n409 = Delete(path (use dialog)=w1027) -> (error out=w1026:errorcluster)  [unwired: 1 in, 5 out]
    }
  }
  n410 = Close Reference(reference=w12) -> (error out=w6:errorcluster)  [unwired: 1 in]
  n411 = Close Reference(reference=w13) -> (error out=w7:errorcluster)  [unwired: 1 in]
  n412 = Close Reference(reference=w11) -> (error out=w5:errorcluster)  [unwired: 1 in]
  n413 = Close Reference(reference=w14) -> (error out=w8:errorcluster)  [unwired: 1 in]
  n414 = Close Reference(reference=w15) -> ()  [unwired: 1 in, 1 out]
  n415 = Close Reference(reference=w23) -> (error out=w10:errorcluster)  [unwired: 1 in]
  n416 = Close Reference(reference=w26) -> (error out=w9:errorcluster)  [unwired: 1 in]
  n417 = stacked-sequence {
    tunnel: w10 -> [w1028]
    tunnel: w9 -> [_]
    tunnel: w8 -> [_]
    tunnel: w7 -> [_]
    tunnel: w6 -> [_]
    tunnel: w5 -> [_]
    tunnel: w4 -> [w1029]
    tunnel: [w1028] -> w3
    frame #0 {
      n418 = Close Reference(reference=w1029) -> ()  [unwired: 1 in, 1 out]
    }
  }
  n419 = stacked-sequence {
    tunnel: w19 -> [w1033]
    tunnel: [FALSE ("Front Panel Window:Open")] -> w16
    tunnel: w3 -> [_]
    tunnel: [w1031] -> _
    tunnel: [w1030] -> _
    frame #0 {
      n420 = call <vilib>:"Unset Busy.vi"() -> ()  [unwired: 2 in, 10 out]
      n421 = invoke on="Attribute Before" class="SubPanel" method="Remove VI"() -> (error out=w1031:errorcluster)  [unwired: 3 in, 2 out]
      n422 = invoke on="Attribute After" class="SubPnl" method="Remove VI"() -> (error out=w1030:errorcluster)  [unwired: 3 in, 2 out]
      "Cancel" <- w1033
    }
  }
  n423 = property class="VI"("Front Panel Window:Open"=w16) -> ()  [unwired: 2 in, 2 out]
